vi "FA_WC_Divisions.vi"() -> ()   [LabVIEW 2013]
uses:
  FA_LocalStore API/source/VI Source/FA_LSSpecialTypes.ctl
  <vilib>/Utility/file.llb/Read From Spreadsheet File (string).vi
  FA_LocalStore API/source/VI Source/FA_LocalStore.lvlib
  <vilib>/Utility/file.llb/Write To Spreadsheet File (string).vi
panel:
  out "all rows":string[][](array[string])
  in  "Attendance Debug":string[][](array[string])=array400x82[32800 elements]
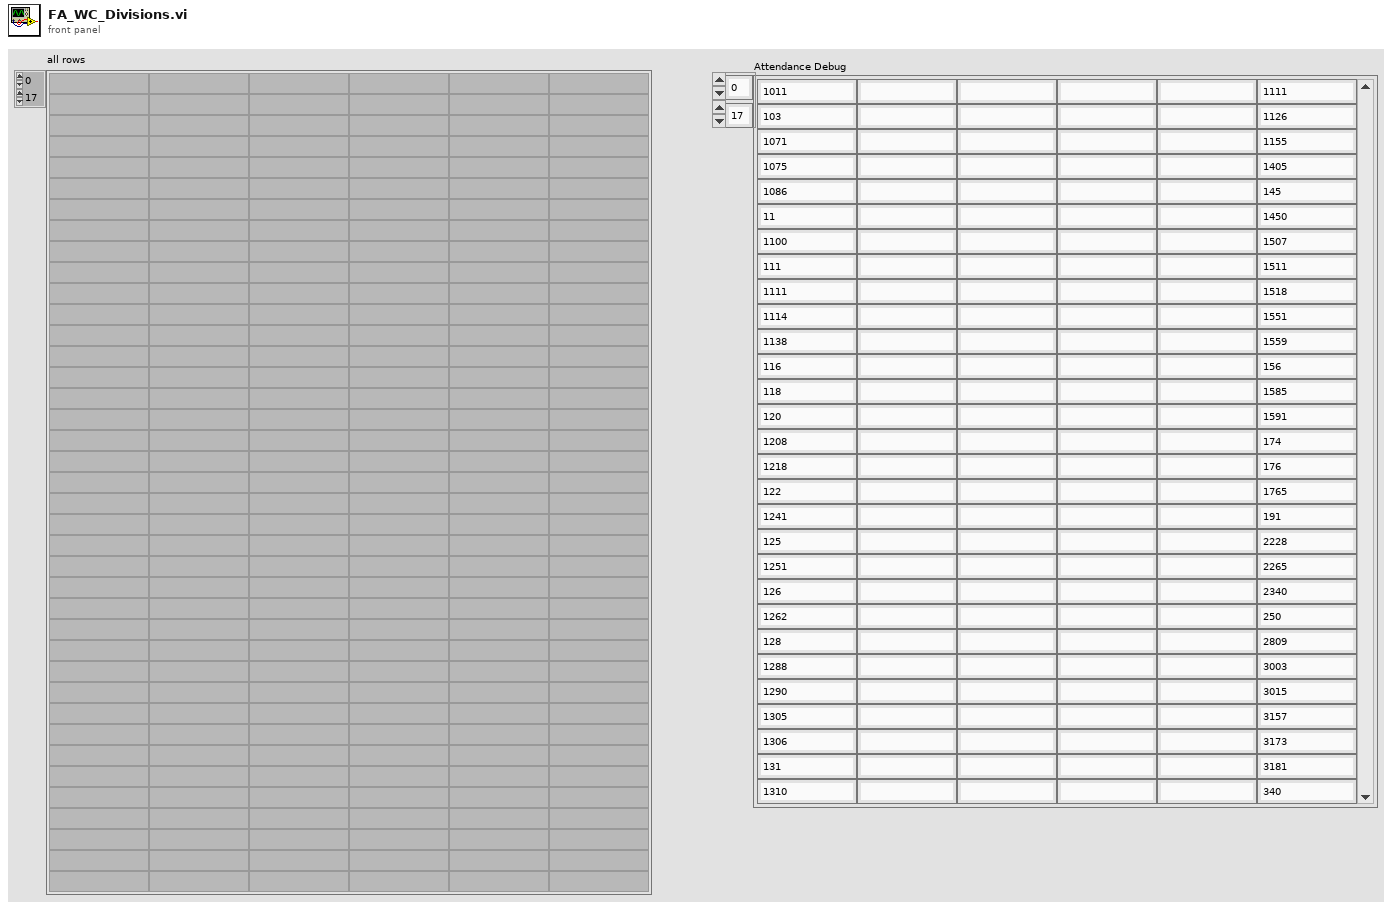
[diagram p1: front panel]
types:
  T1 = typedef "FA_LocalStore.lvlib/FA_LSSpecialTypes.ctl" = string
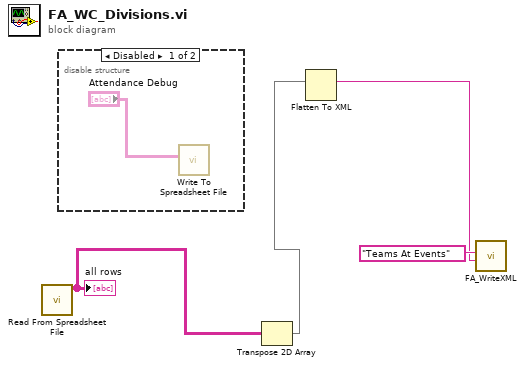
[diagram p0: block diagram]
diagram:
  n1 = call-poly <vilib>:"Read From Spreadsheet File.vi"() -> ("all rows"=w2:string[][])  [unwired: 7 in, 4 out]
  "all rows" <- w2
  n2 = disable-structure shown="Disabled" {
    frame Disabled {
      n3 = call-poly <vilib>:"Write To Spreadsheet File.vi"("2D data"="Attendance Debug") -> ()  [unwired: 7 in, 1 out]
    }
    frame Enabled {
    }
  }
  n4 = Transpose 2D Array(2D array=w2) -> (transposed array=w1:string[][])
  n5 = Flatten To XML(anything=w1) -> (xml string=w3:string)
  n6 = call "FA_WriteXML.vi"("XML String"=w3, "Special Type"=T1 "Teams At Events") -> ()  [unwired: 7 in, 1 out]
